vi "I2S Clock(David Documentation).vi"(8 "I2S.BitCount":u16=31, 11 "I2S.MCLK":bool) -> (2 "I2S.PBLRC/RECLRC OUT":bool, 3 "I2S.BCLK OUT":bool)   [LabVIEW 2015]
panel:
  # "Overviews: Clock Derivation from MCKL signal. Output Clock Signals are: BCLK, PBLRC and RECLRC."
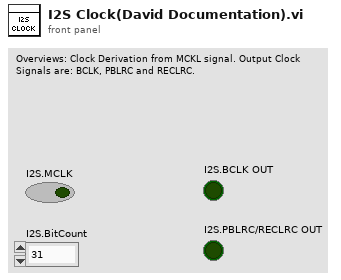
[diagram p1: front panel]
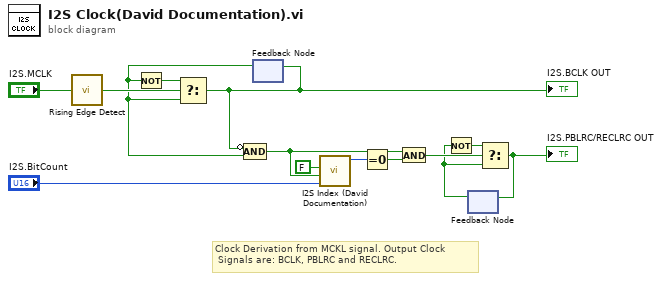
[diagram p0: block diagram]
diagram:
  # "Clock Derivation from MCKL signal. Output Clock\n Signals are: BCLK, PBLRC and RECLRC."
  n1 = call "Rising Edge Detect.vi"("Signal"="I2S.MCLK") -> ("Trigger?"=w12:bool)
  n2 = feedback #1() -> (w10:bool)  [unwired: 1 in]
  n3 = Not(x=w10) -> (.not. x?=w13:bool)
  n4 = Select(t=w13, s=w12, f=w10) -> (s? t:f=w11:bool)
  "I2S.BCLK OUT" <- w11
  n5 = Compound Arithmetic op=AND(invert w11, w10) -> (w2:bool)
  n6 = feedback-in #1(w11) -> ()
  n7 = call "I2S Index (David Documentation).vi"("Bit Count"="I2S.BitCount", "Update"=w2, "Change Channel"=FALSE) -> ("Value Out"=w4:u16)  [unwired: 8 in]
  n8 = Equal To 0?(x=w4) -> (x = 0?=w1:bool)
  n9 = And(x=w2, y=w1) -> (x .and. y?=w6:bool)
  n10 = feedback #2() -> (w5:bool)  [unwired: 1 in]
  n11 = Not(x=w5) -> (.not. x?=w7:bool)
  n12 = Select(t=w7, s=w6, f=w5) -> (s? t:f=w3:bool)
  "I2S.PBLRC/RECLRC OUT" <- w3
  n13 = feedback-in #2(w3) -> ()
